vi "Set Default Drop-In.vi"() -> (0 "error out":errorcluster)   [LabVIEW 2016]
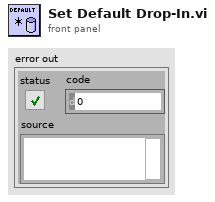
[diagram p1: front panel]
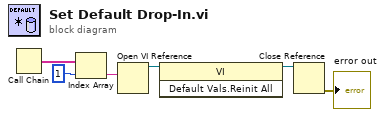
[diagram p0: block diagram]
diagram:
  n1 = Call Chain() -> (call chain=w6:string[])
  n2 = Index Array(array=w6, index=1) -> (element=w4:string)
  n3 = Open VI Reference(vi path=w4) -> (vi reference=w3:refnum<vi>)  [unwired: 5 in, 1 out]
  n4 = invoke class="VI" method="Default Vals.Reinit All"(reference=w3) -> (reference out=w2:refnum<vi>)  [unwired: 2 in, 2 out]
  n5 = Close Reference(reference=w2) -> (error out=→"error out":errorcluster)  [unwired: 1 in]
